vi "exampleWriteToMyRIO.vi"() -> ()   [LabVIEW 2019]
panel:
  out "error out 2":errorcluster caption="error out"
  in  "file path (use dialog)":path
  out "error out":errorcluster
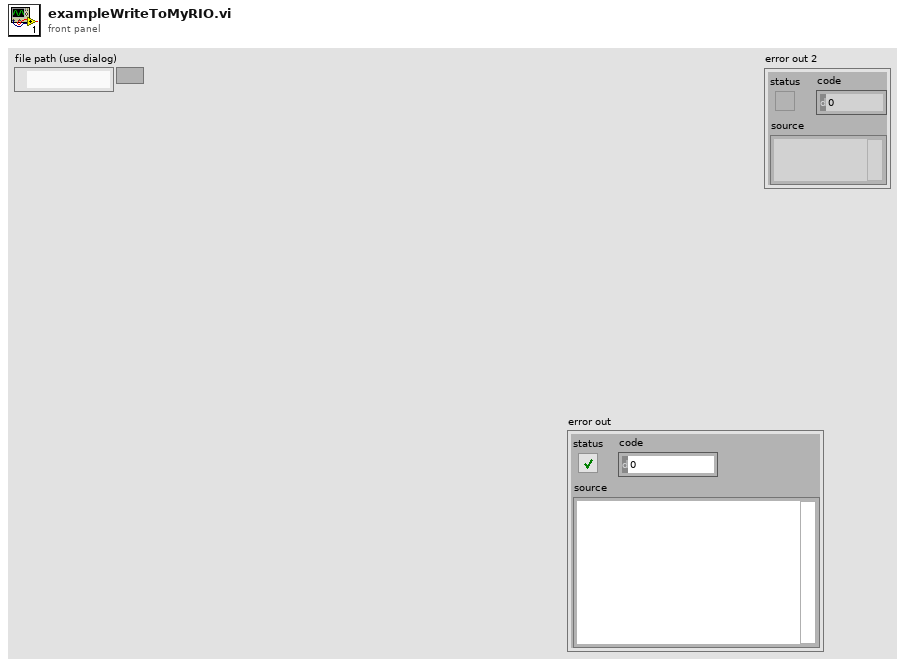
[diagram p1: front panel]
types:
  T1 = enum16{"open", "replace", "create", "open or create", "replace or create", "replace or create with confirmation"}
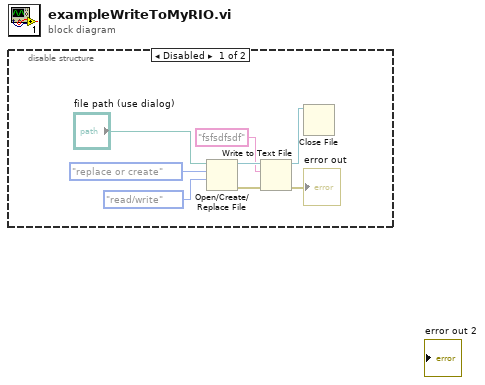
[diagram p0: block diagram]
diagram:
  n1 = disable-structure shown="Disabled" {
    frame Disabled {
      n2 = Open/Create/Replace File(file path (use dialog)="file path (use dialog)", operation (0:open)=T1."replace or create", access (0:read/write)=enum16{"read/write", "read-only", "write-only"}."read/write") -> (refnum out=w4:refnum<file>, error out=w7:errorcluster)  [unwired: 3 in, 1 out]
      n3 = Write to Text File(file (use dialog)=w4, text="fsfsdfsdf", error in=w7) -> (refnum out=w3:refnum<file>, error out=→"error out":errorcluster)  [unwired: 1 in, 1 out]
      n4 = Close File(refnum=w3) -> ()  [unwired: 1 in, 2 out]
    }
    frame Enabled {
    }
  }
